vi "GUI_Bella_BTLsmall_nocams.vi"() -> ()   [LabVIEW 2020]
uses:
  Device Drivers/LEPS Interface/Filter_typdef.ctl
  Shared/GUI_Template/GUI_master/tcp_new_data_event.ctl
  Shared/GUI_Template/GUI_master/tcp new data cluster.ctl
  GUI_TestStand/Fire button.ctl
  Device Drivers/DG645/subVIs/TriggerSource_TypDef.ctl
panel:
  in  "Stepsize":dbl=0.001 caption="Step Size" min=0.0 max=1.0 format="%.3f"
  in  "Trigger.Source::10":T1=enum."External rising edges" caption="SRS Trigger Mode"
  in  "relativeMove.Axis 2neg::6":bool
  in  "relativeMove.Axis 2pos::6":bool
  in  "relativeMove.Axis 3pos::6":bool
  in  "relativeMove.Axis 3neg::6":bool
  out "fire::10":string="fire" caption="fire"
  in  "GUIdevice 10":string="DDG-AA-ShotCntrl"
  in  "Fire Button":T2
  in  "relativeMove.Axis 1neg::8":bool
  in  "relativeMove.Axis 1pos::8":bool
  in  "relativeMove.Axis 2pos::8":bool
  in  "relativeMove.Axis 2neg::8":bool
  in  "filter.var 2::9":T3=enum."Open(6)" caption="Filter Wheel"
  out "GUIdevice 5":string="M2Cam"
  in  "relativeMove.Axis 1neg::7":bool
  in  "relativeMove.Axis 1pos::7":bool
  in  "relativeMove.Axis 2pos::7":bool
  in  "relativeMove.Axis 2neg::7":bool
  in  "filter.var 4::9":T3=enum."Open(6)" caption="Filter Wheel"
  out "GUIdevice 3":string="M4Cam"
  in  "centroidx::1":dbl caption="X" min=0.0 max=0.0
  in  "centroidy::1":dbl caption="Y" min=0.0 max=0.0
  in  "filter.var 1::9":T3=enum."Open(6)" caption="Filter Wheel"
  out "GUIdevice 1":string="M1Cam"
  in  "relativeMove.Axis 1pos::6":bool
  in  "relativeMove.Axis 1neg::6":bool
  in  "relativeMove.Axis 3pos::7":bool
  in  "relativeMove.Axis 3neg::7":bool
  out "GUIdevice 2":string="M5Cam"
  in  "filter.var 5::9":T3=enum."Open(6)" caption="Filter Wheel"
  out "stepsize::6":dbl=0.01 caption="Step Size" min=0.0 max=1.0 format="%.3f"
  out "stepsize::7":dbl=0.01 caption="Step Size" min=0.0 max=1.0 format="%.3f"
  out "stepsize::8":dbl=0.01 caption="Step Size" min=0.0 max=1.0 format="%.3f"
  in  "GUIdevice 9":string="71146 LEPS Interface"
  out "tcp data event":T4
  in  "GUIdevice 8":string="MCD-1BL-ESP301M1"
  in  "GUIdevice 7":string="MCD-1BL-ESP301M2M4"
  in  "GUIdevice 6":string="MCD-1BL-ESP301M4M5"
  in  "stop":bool
  out "error IO 2":errorcluster
  # "Arrows move mirror associated with it.\nFilters apply to camera looking at that mirror."
  # "Centroid"
  # "M5 X-Axis, LP Mode CAMS"
  # "M5 Y-Axis, M4 CAMS"
  # "M2 CAM"
  # "M5 and LP Mode CAMS"
  # "M4 and M5 CAMS"
  # "M2 CAM"
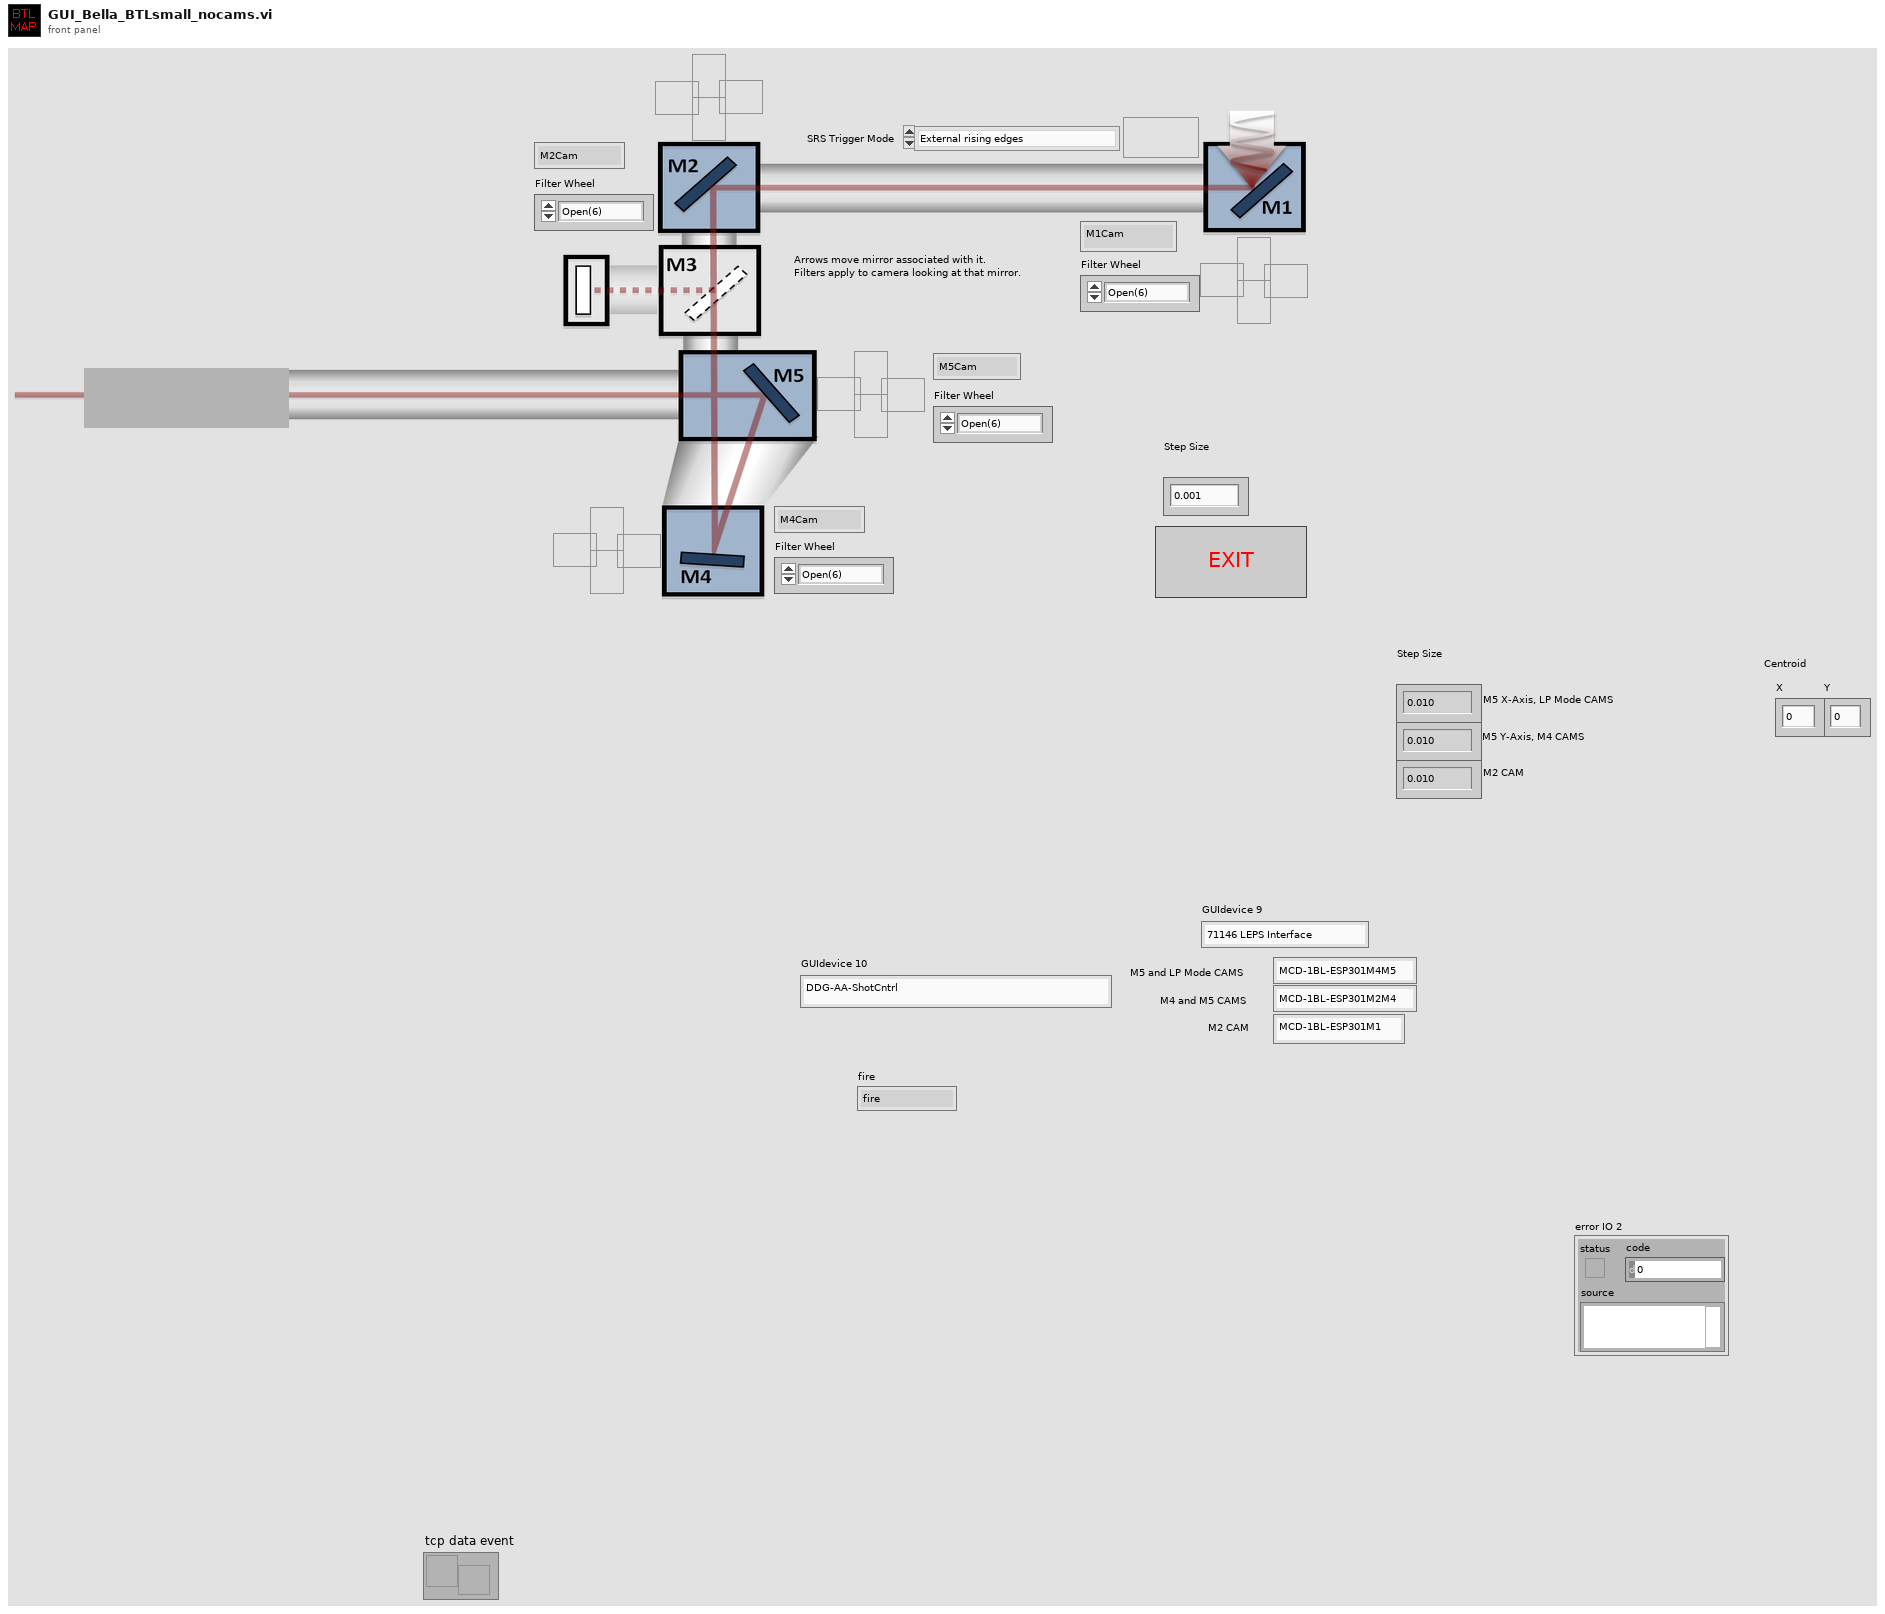
[diagram p1: front panel]
types:
  T1 = typedef "TriggerSource_TypDef.ctl" = enum16{"Internal", "External rising edges", "External falling edges", "Single shot external rising edges", "Single shot external falling edges", "Single shot", "Line"}
  T2 = typedef "Fire button.ctl" = bool
  T3 = typedef "Filter_typdef.ctl" = enum16{"Moving/Unknown", "OD1", "OD2", "OD3", "OD4", "OD5", "Open(6)"}
  T4 = typedef "tcp_new_data_event.ctl" = refnum<user-event>
  T5 = typedef "tcp new data cluster.ctl" = cluster{"EventEnum":enum16{"new data", "connection status update"}, "Device name":string}
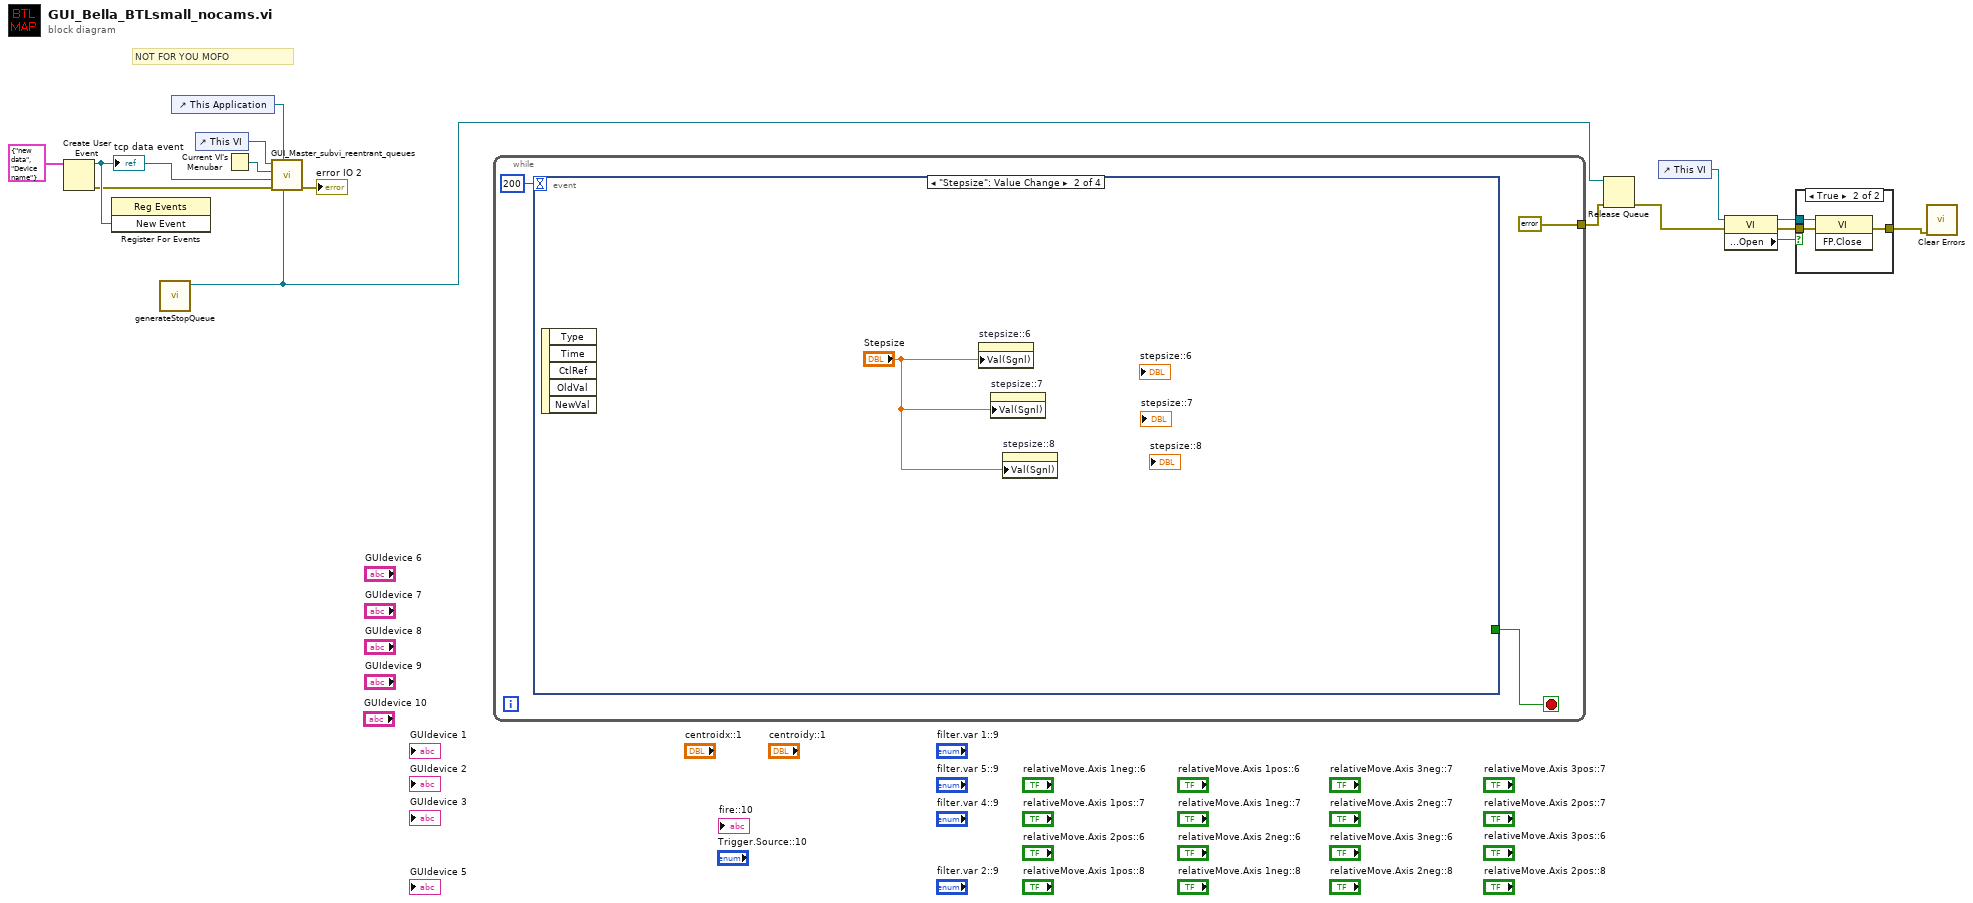
[diagram p0: block diagram]
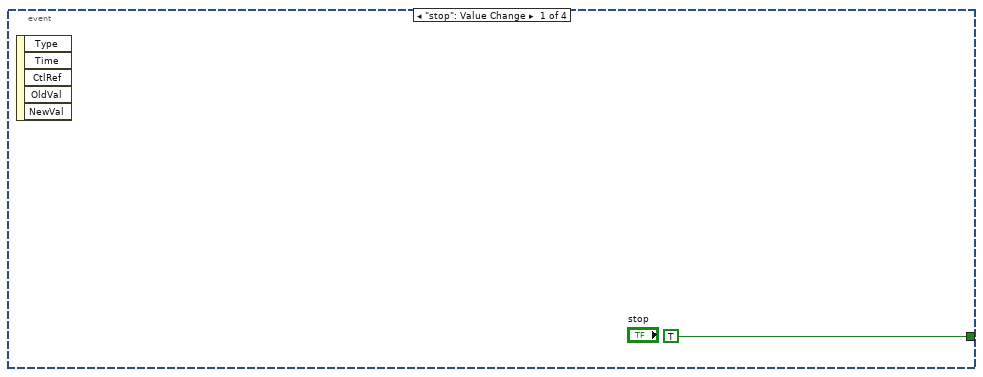
[diagram p3: hidden frame]
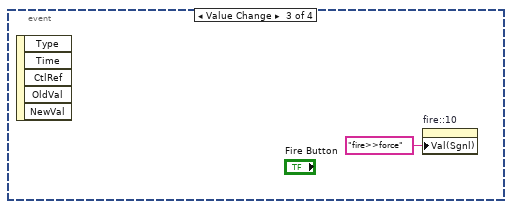
[diagram p4: hidden frame]
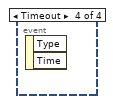
[diagram p5: hidden frame]
diagram:
  # "NOT FOR YOU MOFO"
  n1 = Create User Event(user event datatype=T5 {"EventEnum"=enum."new data", "Device name"="Device name"} ("New Event")) -> (user event=w14:refnum<user-event>, error out=w13:errorcluster)  [unwired: 1 in]
  "tcp data event" <- w14
  n2 = register-events(w14) -> ()  [unwired: 2 in, 2 out]
  n3 = call "generateStopQueue.vi"() -> ("STOP Queue out"=w8:refnum<queue>)  [unwired: 10 in, 1 out]
  n4 = control-ref of="This Application"() -> (w15:refnum<vi>)
  n5 = control-ref of="This VI"() -> (w10:refnum<vi>)
  n6 = Current VI's Menubar() -> (w11:refnum<k9>)
  n7 = call "GUI_Master_subvi_reentrant_queues.vi"("STOP Queue in"=w8, "This Application"=w15, "error in (no error)"=w13, "tcp data event"=w14, "Caller menu reference"=w11, "Caller VI ref"=w10) -> ("error out"=→"error IO 2":errorcluster)  [unwired: 5 in]
  n8 = while {
    tunnel: [errorcluster {"status"=FALSE, "code"=0, "source"=""} ("error in (no error)")] -> w7
    stop <- w18 stop-if-true
    n9 = event shown="[1] \"Stepsize\": Value Change" {
      selector: _ -> [_ _ _ _]
      dyn-events: _ -> [_ _ _ _]
      timeout: 200 -> [_ _ _ _]
      tunnel: [TRUE ("stop") _ _ _] -> w18
      event "stop": Value Change {
        n10 = event-data() -> ()  [unwired: 1 in, 5 out]
      }
      event "Stepsize": Value Change {
        n11 = event-data() -> ()  [unwired: 1 in, 5 out]
        n12 = property on="stepsize::6" class="DigNum (strict)"("Val(Sgnl)"="Stepsize") -> ()  [unwired: 2 in, 2 out]
        n13 = property on="stepsize::7" class="DigNum (strict)"("Val(Sgnl)"="Stepsize") -> ()  [unwired: 2 in, 2 out]
        n14 = property on="stepsize::8" class="DigNum (strict)"("Val(Sgnl)"="Stepsize") -> ()  [unwired: 2 in, 2 out]
      }
      event Value Change {
        n15 = event-data() -> ()  [unwired: 1 in, 5 out]
        n16 = property on="fire::10" class="Str"("Val(Sgnl)"="fire>>force" ("Value (Signaling)")) -> ()  [unwired: 2 in, 2 out]
      }
      event Timeout {
        n17 = event-data() -> ()  [unwired: 1 in, 2 out]
      }
    }
  }
  n18 = Release Queue(queue=w8, error in (no error)=w7) -> (error out=w2:errorcluster)  [unwired: 1 in, 2 out]
  n19 = control-ref of="This VI"() -> (w3:refnum<vi>)
  n20 = property class="VI"(reference=w3, error in=w2) -> (reference out=w5:refnum<vi>, error out=w6:errorcluster, "Front Panel.Open"=w4:bool)
  n21 = case shown="True" w4 {
    tunnel: [w22 w25] -> w1
    tunnel: w6 -> [w22 w24]
    tunnel: w5 -> [_ w23]
    frame False {
    }
    frame True {
      n22 = invoke class="VI" method="FP.Close"(reference=w23, error in=w24) -> (error out=w25:errorcluster)  [unwired: 1 in, 2 out]
    }
  }
  n23 = call <vilib>:"Clear Errors.vi"("error in (no error)"=w1) -> ()  [unwired: 5 in, 2 out]
